vi "Teleop.vi"(10 "Match Info":T1={"Autonomous Elapsed Seconds"=0.0, "TeleOp Elapsed Seconds"=0.0, "Disabled Elapsed Seconds"=0.0, "Visited Autonomous"=FALSE, "Visited TeleOp"=FALSE, "Visited Disabled"=FALSE, "Autonomous Settings"={"Autonomous Style"=enum."Independent", "VI Refnum"=refnum}}, 11 "Call Context":T2) -> ()   [LabVIEW 2020]
doc: "This VI is called for each TeleOp packet received from the DS where the robot is not disabled. It is often used to read from the joysticks and update I/O or to update setpoints for timed control loops. It should complete and return within 20 milliseconds or it may miss DS packets."
uses:
  <vilib>/Rock Robotics/WPI/DriverStation/WPI_DriverStationDerivedRobotMode.ctl
  <vilib>/Rock Robotics/WPI/DriverStation/WPI_DriverStationMatch Info.ctl
  <vilib>/Rock Robotics/WPI/Utilities/WPI_GetSetVariantRefNum.vi
  2017 Swerve Code/Swerve Global Variables.vi
  Robot Global Data.vi
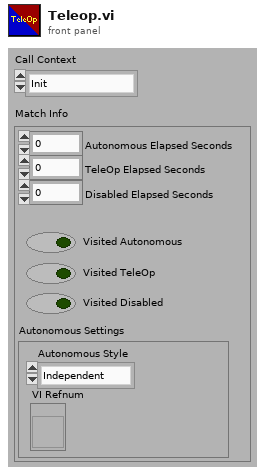
[diagram p1: front panel]
types:
  T1 = typedef "WPI_DriverStationMatch Info.ctl" = cluster{"Autonomous Elapsed Seconds":dbl, "TeleOp Elapsed Seconds":dbl, "Disabled Elapsed Seconds":dbl, "Visited Autonomous":bool, "Visited TeleOp":bool, "Visited Disabled":bool, "Autonomous Settings":cluster{"Autonomous Style":enum16{"Iterative", "Independent"}, "VI Refnum":refnum<vi>}}
  T2 = typedef "WPI_DriverStationDerivedRobotMode.ctl" = enum16{"Init", "Execute", "Stop"}
  T3 = typedef "WPI_JoystickDevRef.ctl" = cluster{"Device":T4}
  T4 = typedef "WPI_JoystickDeviceEnum.ctl" = enum16{"USB 0", "USB 1", "USB 2", "USB 3", "USB 4", "USB 5"}
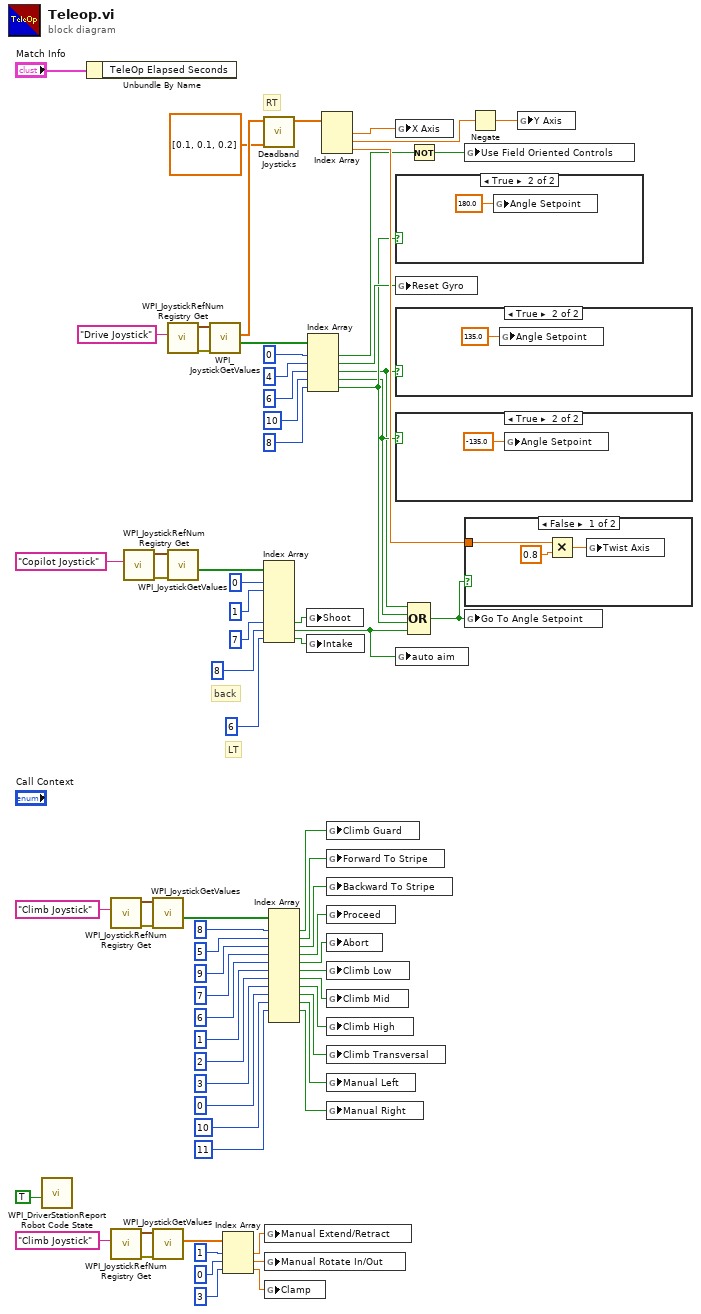
[diagram p0: block diagram]
diagram:
  # "RT"
  # "back"
  # "LT"
  n1 = call <vilib>:"WPI_DriverStationReport Robot Code State.vi"("TeleOp"=TRUE ("Autonomous")) -> ()  [unwired: 10 in, 1 out]
  n2 = Unbundle By Name("Match Info") -> ()  [unwired: 1 out]
  n3 = call <vilib>:"WPI_JoystickRefNum Registry Get.vi"("refnum name"="Climb Joystick") -> ("error out"=w45:errorcluster, "JoystickDevRef"=w44:T3)  [unwired: 9 in]
  n4 = call <vilib>:"WPI_JoystickRefNum Registry Get.vi"("refnum name"="Climb Joystick") -> ("error out"=w42:errorcluster, "JoystickDevRef"=w41:T3)  [unwired: 9 in]
  n5 = call <vilib>:"WPI_JoystickRefNum Registry Get.vi"("refnum name"="Copilot Joystick") -> ("error out"=w55:errorcluster, "JoystickDevRef"=w56:T3)  [unwired: 1 in, 8 out]
  n6 = call <vilib>:"WPI_JoystickGetValues.vi"("error in (no error)"=w45, "JoystickDevRef"=w44) -> ("Buttons"=w38:bool[])  [unwired: 5 in, 4 out]
  n7 = call <vilib>:"WPI_JoystickGetValues.vi"("error in (no error)"=w42, "JoystickDevRef"=w41) -> ("Axes"=w39:dbl[])  [unwired: 5 in, 4 out]
  n8 = call <vilib>:"WPI_JoystickRefNum Registry Get.vi"("refnum name"="Drive Joystick") -> ("error out"=w61:errorcluster, "JoystickDevRef"=w71:T3)  [unwired: 1 in, 8 out]
  n9 = call <vilib>:"WPI_JoystickGetValues.vi"("error in (no error)"=w55, "JoystickDevRef"=w56) -> ("Buttons"=w54:bool[])  [unwired: 5 in, 4 out]
  n10 = call <vilib>:"WPI_JoystickGetValues.vi"("error in (no error)"=w61, "JoystickDevRef"=w71) -> ("Buttons"=w65:bool[], "Axes"=w60:dbl[])  [unwired: 5 in, 3 out]
  n11 = Index Array(array=w39, index #1=1 ("index"), index #2=0 ("index"), index #3=3 ("index")) -> (element #1=w14:dbl, element #2=w13:dbl, element #3=w10:dbl)
  n12 = call "Deadband Joysticks.vi"("Deadbands"=dbl[] [0.1, 0.1, 0.2], "Axes"=w60) -> ("Axes'"=w58:dbl[])  [unwired: 9 in]
  n13 = Index Array(array=w54, index #1=0 ("index"), index #2=1 ("index"), index #6=7 ("index"), index #7=8 ("index"), index #8=6 ("index")) -> (element #6=w46:bool, element #7=w6:bool, element #8=w48:bool)  [unwired: 3 in, 5 out]
  n14 = global write "Swerve Global Variables.vi" "Manual Extend/Retract"(w14) -> ()
  n15 = global write "Swerve Global Variables.vi" "Manual Rotate In/Out"(w13) -> ()
  n16 = global write "Swerve Global Variables.vi" "Clamp"(w10) -> ()
  n17 = Index Array(array=w38, index #1=8 ("index"), index #2=5 ("index"), index #3=9 ("index"), index #4=7 ("index"), index #5=6 ("index"), index #6=1 ("index"), index #7=2 ("index"), index #8=3 ("index"), index #9=0 ("index"), index #10=10 ("index"), index #11=11 ("index")) -> (element #1=w37:bool, element #2=w34:bool, element #3=w33:bool, element #4=w31:bool, element #5=w29:bool, element #6=w27:bool, element #7=w25:bool, element #8=w23:bool, element #9=w21:bool, element #10=w19:bool, element #11=w17:bool)  [unwired: 1 in, 1 out]
  n18 = global write "Robot Global Data.vi" "Shoot"(w46) -> ()
  n19 = global write "Robot Global Data.vi" "Intake"(w48) -> ()
  n20 = Index Array(array=w65, index #1=0 ("index"), index #2=4 ("index"), index #3=6 ("index"), index #4=10 ("index"), index #5=8 ("index")) -> (element #1=w64:bool, element #2=w62:bool, element #3=w3:bool, element #4=w4:bool, element #5=w5:bool)
  n21 = Index Array(array=w58) -> (element #1=w69:dbl, element #2=w68:dbl, element #3=w67:dbl)  [unwired: 3 in]
  n22 = global write "Robot Global Data.vi" "Climb Guard"(w37) -> ()
  n23 = global write "Robot Global Data.vi" "Forward To Stripe"(w34) -> ()
  n24 = global write "Robot Global Data.vi" "Backward To Stripe"(w33) -> ()
  n25 = global write "Robot Global Data.vi" "Proceed"(w31) -> ()
  n26 = global write "Robot Global Data.vi" "Abort"(w29) -> ()
  n27 = global write "Robot Global Data.vi" "Climb Low"(w27) -> ()
  n28 = global write "Robot Global Data.vi" "Climb Mid"(w25) -> ()
  n29 = global write "Robot Global Data.vi" "Climb High"(w23) -> ()
  n30 = global write "Robot Global Data.vi" "Climb Transversal"(w21) -> ()
  n31 = global write "Robot Global Data.vi" "Manual Left"(w19) -> ()
  n32 = global write "Robot Global Data.vi" "Manual Right"(w17) -> ()
  n33 = global write "Swerve Global Variables.vi" "X Axis"(w69) -> ()
  n34 = case shown="True" w5 {
    frame False {
    }
    frame True {
      n35 = global write "Robot Global Data.vi" "Angle Setpoint"(180.0 ("Angle Setpoint")) -> ()
    }
  }
  n36 = global write "Swerve Global Variables.vi" "Reset Gyro"(w62) -> ()
  n37 = case shown="True" w3 {
    frame False {
    }
    frame True {
      n38 = global write "Robot Global Data.vi" "Angle Setpoint"(135.0 ("Angle Setpoint")) -> ()
    }
  }
  n39 = case shown="True" w4 {
    frame False {
    }
    frame True {
      n40 = global write "Robot Global Data.vi" "Angle Setpoint"(-135.0 ("Angle Setpoint")) -> ()
    }
  }
  n41 = global write "Robot Global Data.vi" "auto aim"(w6) -> ()
  n42 = Compound Arithmetic op=OR(w3, w4, w5, w6) -> (w2:bool)
  n43 = Not(x=w64) -> (.not. x?=w63:bool)
  n44 = global write "Swerve Global Variables.vi" "Use Field Oriented Controls"(w63) -> ()
  n45 = case shown="False" w2 {
    tunnel: w67 -> [w79 _]
    frame False {
      n46 = Multiply(x=w79, y=0.8) -> (x*y=w78:dbl)
      n47 = global write "Swerve Global Variables.vi" "Twist Axis"(w78) -> ()
    }
    frame True {
    }
  }
  n48 = global write "Robot Global Data.vi" "Go To Angle Setpoint"(w2) -> ()
  n49 = Negate(x=w68) -> (-x=w66:dbl)
  n50 = global write "Swerve Global Variables.vi" "Y Axis"(w66) -> ()
